vi "Flash_ADB.vi"() -> (0 "error out":errorcluster, 1 "standard output":string, 3 "Result":bool)   [LabVIEW 2018]
panel:
  out "Return Val":i32
  in  "Path":path=path "C:/ADB_FLASH/MK10_New/adb_mk10_new.bat"
  out "cmd line":string
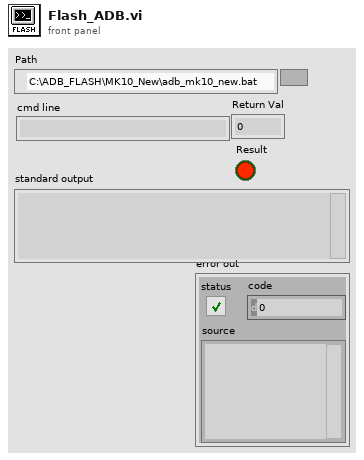
[diagram p1: front panel]
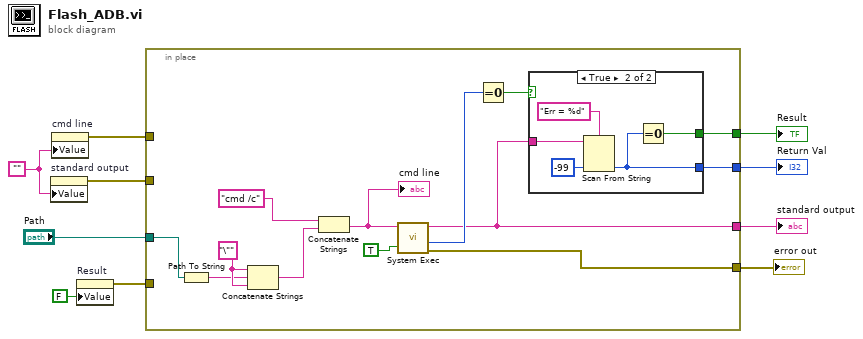
[diagram p0: block diagram]
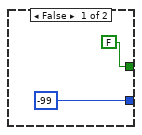
[diagram p2: hidden frame]
diagram:
  w6 = ""
  n1 = property on="standard output" class="Str"("Value"=w6) -> (error out=w7:errorcluster)  [unwired: 2 in, 1 out]
  n2 = property on="cmd line" class="Str"("Value"=w6) -> (error out=w8:errorcluster)  [unwired: 2 in, 1 out]
  n3 = property on="Result" class="Bool (strict)"("Value"=FALSE ("Result")) -> (error out=w10:errorcluster)  [unwired: 2 in, 1 out]
  n4 = in-place {
    in-place-border: w10 -> [_]
    in-place-border: w8 -> [_]
    in-place-border: w7 -> [_]
    in-place-border: [w15] -> w5
    in-place-border: [w16] -> w4
    in-place-border: [w14] -> w3
    in-place-border: [w12] -> w2
    in-place-border: "Path" -> [w11]
    w23 = "\"" ("string")
    n5 = Path To String(path=w11) -> (string=w18:string)
    n6 = Concatenate Strings(w23, w18, w23) -> (w19:string)
    n7 = Concatenate Strings("cmd /c" ("string"), w19) -> (w21:string)
    "cmd line" <- w21
    n8 = call <vilib>:"System Exec.vi"("run minimized? (F)"=TRUE, "command line"=w21) -> ("error out"=w16:errorcluster, "return code"=w17:i32, "standard output"=w15:string)  [unwired: 6 in, 1 out]
    n9 = Equal To 0?(x=w17) -> (x = 0?=w13:bool)
    n10 = case shown="True" w13 {
      tunnel: w15 -> [_ w29]
      tunnel: [-99 ("default value 1") w26] -> w14
      tunnel: [FALSE w27] -> w12
      frame False {
      }
      frame True {
        n11 = Scan From String(format string="Err = %d", input string=w29, default 1=-99 ("default value 1")) -> (output 1=w26:i32)  [unwired: 2 in, 3 out]
        n12 = Equal To 0?(x=w26) -> (x = 0?=w27:bool)
      }
    }
  }
  "Result" <- w2
  "standard output" <- w5
  "error out" <- w4
  "Return Val" <- w3
